vi "EletoMatr.vi"(0 "Input Array X":dbl[][](array[numeric]), 9 "In Row":dbl, 11 "In Column":dbl, 12 "Input Direction":bool=TRUE) -> (3 "Completed":bool=TRUE, 4 "Out Array X":dbl[][](array[numeric]), 10 "Out Row":dbl, 14 "Output Direction":bool=TRUE, 15 "Out Column":dbl)   [LabVIEW 2012]
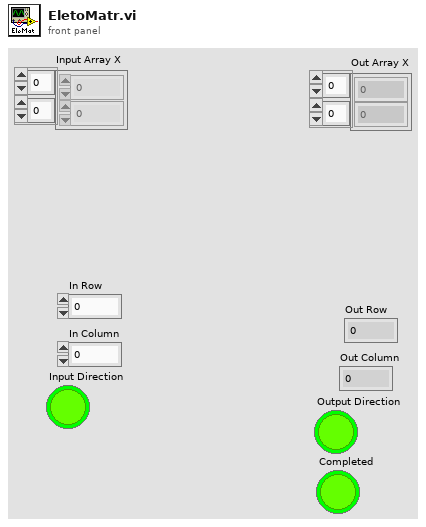
[diagram p1: front panel]
types:
  T1 = typedef "NI_Matrix.lvlib/RealMatrix.ctl" = dbl[][]
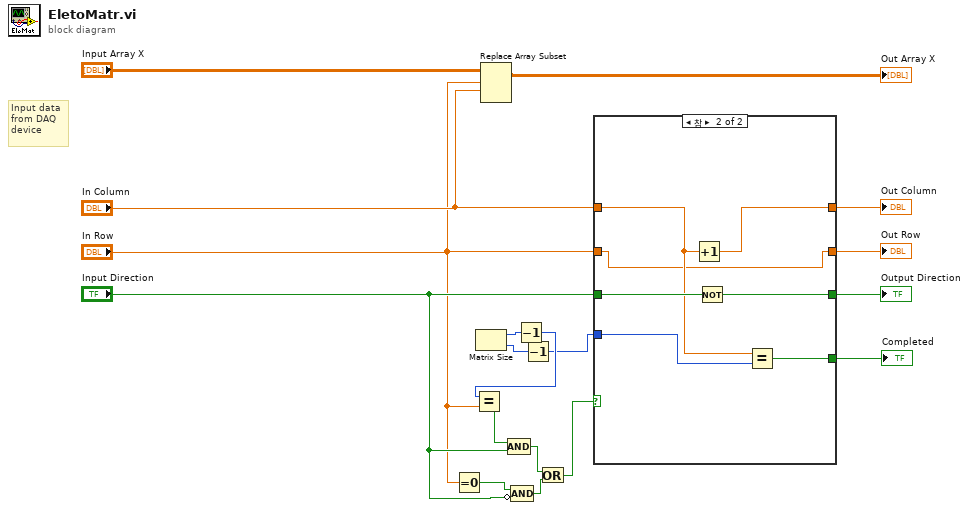
[diagram p0: block diagram]
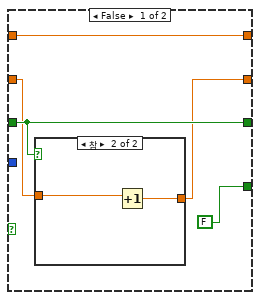
[diagram p2: hidden frame]
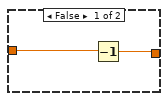
[diagram p3: hidden frame]
diagram:
  # "Input data\nfrom DAQ\ndevice"
  n1 = Equal To 0?(x="In Row") -> (x = 0?=w4:bool)
  n2 = Matrix Size() -> (1:w9:i32, 2:w8:i32)  [unwired: 1 in]
  n3 = Replace Array Subset(array="Input Array X", index (row)="In Row", index (col)="In Column") -> (→"Out Array X":T1)  [unwired: 1 in]
  n4 = Compound Arithmetic op=AND(w4, invert "Input Direction") -> (w11:bool)
  n5 = Decrement(x=w9) -> (x-1=w2:i32)
  n6 = Equal?(x=w2, y="In Row") -> (x = y?=w7:bool)
  n7 = Compound Arithmetic op=AND(w7, "Input Direction") -> (w5:bool)
  n8 = Decrement(x=w8) -> (x-1=w1:i32)
  n9 = Or(x=w5, y=w11) -> (x .or. y?=w10:bool)
  n10 = case shown="참" w10 {
    tunnel: "Input Direction" -> [w23 w34]
    tunnel: "In Row" -> [w21 w28]
    tunnel: [w19 w29] -> w17
    tunnel: "In Column" -> [w19 w30]
    tunnel: [w23 w33] -> w16
    tunnel: [w20 w28] -> w15
    tunnel: w1 -> [_ w31]
    tunnel: [FALSE w32] -> w13
    frame False {
      n11 = case shown="참" w23 {
        tunnel: [w25 w27] -> w20
        tunnel: w21 -> [w24 w26]
        frame False {
          n12 = Decrement(x=w24) -> (x-1=w25:dbl)
        }
        frame True {
          n13 = Increment(x=w26) -> (x+1=w27:dbl)
        }
      }
    }
    frame True {
      n14 = Increment(x=w30) -> (x+1=w29:dbl)
      n15 = Not(x=w34) -> (.not. x?=w33:bool)
      n16 = Equal?(x=w30, y=w31) -> (x = y?=w32:bool)
    }
  }
  "Out Row" <- w15
  "Out Column" <- w17
  "Output Direction" <- w16
  "Completed" <- w13
